vi "GPS -SET Server or Cache.vi"(10 "Mode":T1(ring), 11 ".NET Refnum in":refnum<k24>) -> (3 ".NET Refnum out":refnum<k24>)   [LabVIEW 2019]
uses:
  \\mac\Dropbox/gmap.net/GMAP.NET 8.6/data/GMap.NET.WindowsForms.dll
  data/GMap.NET.WindowsForms.dll
  \\mac\Dropbox/gmap.net/GMAP.NET 8.6/data/GMap.NET.Core.dll
  data/GMap.NET.Core.dll
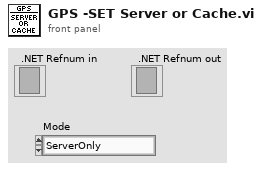
[diagram p1: front panel]
types:
  T1 = enum16{"ServerOnly", "ServerAndCache", "CacheOnly"}
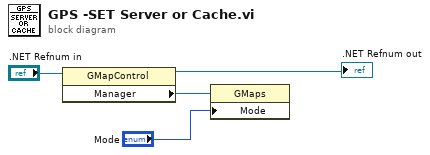
[diagram p0: block diagram]
diagram:
  n1 = property class="GMapControl"(reference=".NET Refnum in") -> (reference out=→".NET Refnum out":refnum<k24>, "Manager"=w2:refnum<k24>)  [unwired: 1 in, 1 out]
  n2 = property class="GMaps"(reference=w2, "Mode"="Mode") -> ()  [unwired: 1 in, 2 out]
